vi "Configure Voltage Protection.vi"(8 "error in (no error)":errorcluster, 9 "Under-Voltage Protection (0.0 V)":dbl min=0.0 max=570.0 format="%.2g", 10 "Over-Voltage Protection (5.0 V)":dbl=5.0 min=0.5 max=650.0 format="%.2g", 11 "VISA resource name":refnum<visa-resource-name>) -> (0 "error out":errorcluster, 3 "VISA resource name out":refnum<visa-resource-name>)   [LabVIEW 2014, in "Agilent N87XX Series.lvlib"]
doc: "Configures over voltage protection (OVP) and under voltage protection (UVP) of the power supply. If the instrument goes outside these limits, then it will disable output. You can monitor this with the Output Protection Status VI."
uses:
  Agilent N87XX Series.lvlib
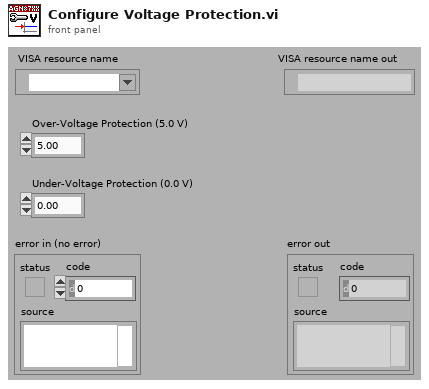
[diagram p1: front panel]
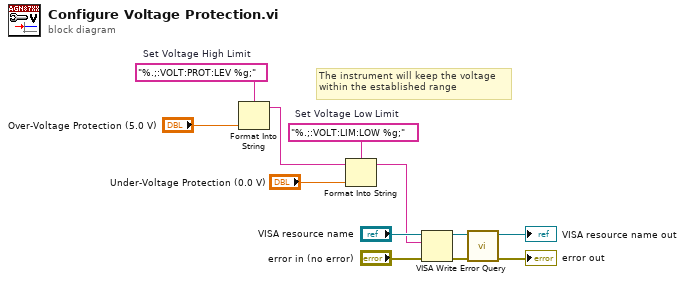
[diagram p0: block diagram]
diagram:
  w4 = "%.;:VOLT:LIM:LOW %g;"  # Set Voltage Low Limit
  w6 = "%.;:VOLT:PROT:LEV %g;"  # Set Voltage High Limit
  # "The instrument will keep the voltage\nwithin the established range"
  n1 = Format Into String(format string=w6, "Over-Voltage Protection (5.0 V)") -> (resulting string=w2:string)  [unwired: 2 in, 1 out]
  n2 = Format Into String(format string=w4, initial string=w2, "Under-Voltage Protection (0.0 V)") -> (resulting string=w1:string)  [unwired: 1 in, 1 out]
  n3 = VISA Write(VISA resource name="VISA resource name", write buffer=w1, error in (no error)="error in (no error)") -> (VISA resource name out=w9:refnum<visa-resource-name>, error out=w10:errorcluster)  [unwired: 1 out]
  n4 = call "Error Query.vi"("error in (no error)"=w10, "VISA resource name"=w9) -> ("error out"=→"error out":errorcluster, "VISA resource name out"=→"VISA resource name out":refnum<visa-resource-name>)  [unwired: 6 in, 2 out]
